vi "aveDirectino.vi"(8 "upper limit":dbl, 9 "upper limit 3":dbl, 10 "upper limit 2":dbl, 11 "upper limit 4":dbl) -> (3 "Numeric":dbl)   [LabVIEW 2014]
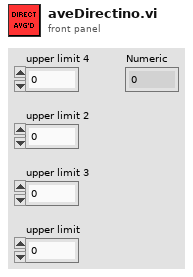
[diagram p1: front panel]
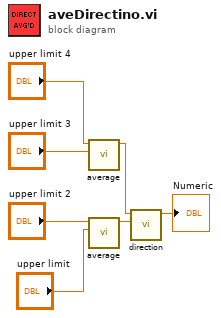
[diagram p0: block diagram]
diagram:
  n1 = call "average.vi"("Numeric in"="upper limit 3", "Numeric 3"="upper limit 4") -> ("Numeric out"=w5:dbl)  [unwired: 9 in]
  n2 = call "average.vi"("Numeric in"="upper limit", "Numeric 3"="upper limit 2") -> ("Numeric out"=w6:dbl)  [unwired: 9 in]
  n3 = call "direction.vi"("upper limit"=w6, "upper limit 2"=w5) -> ("Numeric"=→"Numeric":dbl)  [unwired: 9 in]
